vi "save_processed_data.vi"(8 "error in":errorcluster, 9 "Variable Names Array":string[](array[string]), 10 "variable values":dbl[][](array[numeric]), 11 "base path":path) -> (0 "error out":errorcluster)   [LabVIEW 2013]
doc: "Takes in a 2D string array and save the first column to a \"Processed Data.txt\" file, for use as axes labels by the analysis software."
uses:
  <vilib>/Utility/file.llb/Write To Spreadsheet File (string).vi
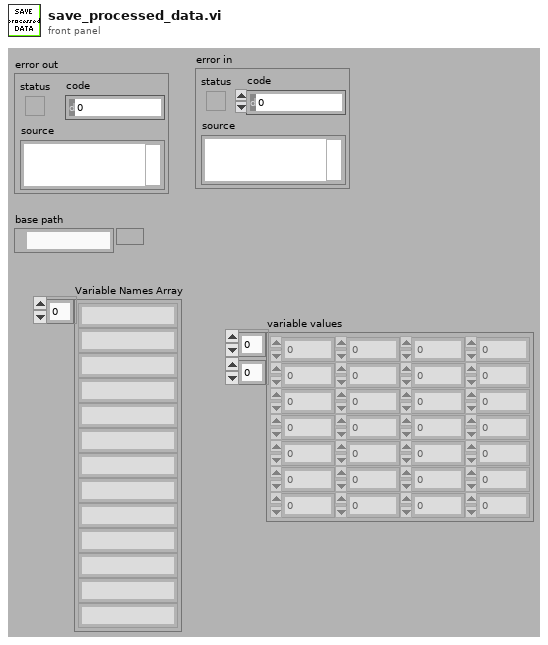
[diagram p1: front panel]
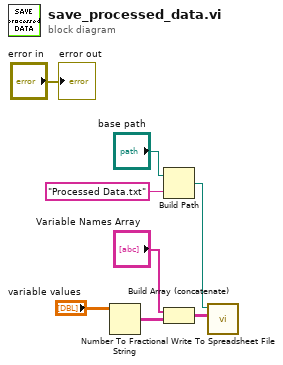
[diagram p0: block diagram]
diagram:
  n1 = Number To Fractional String(number="variable values") -> (F-format string=w3:string[][])  [unwired: 3 in]
  n2 = Build Path(base path="base path", name or relative path="Processed Data.txt") -> (appended path=w5:path)
  n3 = Build Array (concatenate)("Variable Names Array", w3) -> (w1:string[][])
  n4 = call-poly <vilib>:"Write To Spreadsheet File.vi"("2D data"=w1, "file path (dialog if empty)"=w5) -> ()  [unwired: 6 in, 1 out]
  "error out" <- "error in"
